vi "F5xxx_pq_set_harmonics.vi"(7 "max harms":i32=15, 8 "error in":errorcluster, 9 "channel":enum16{"PRI", "SEC"}(ring), 10 "harmonic list":T1[](array[typedef]), 11 "VISA in":refnum<visa-resource-name>) -> (0 "error out":errorcluster, 3 "VISA out":refnum<visa-resource-name>)   [LabVIEW 2013]
uses:
  F5xxx_pq_harmonic_def.ctl
  Fluke 5XXX Series Multicalibrators.lvlib
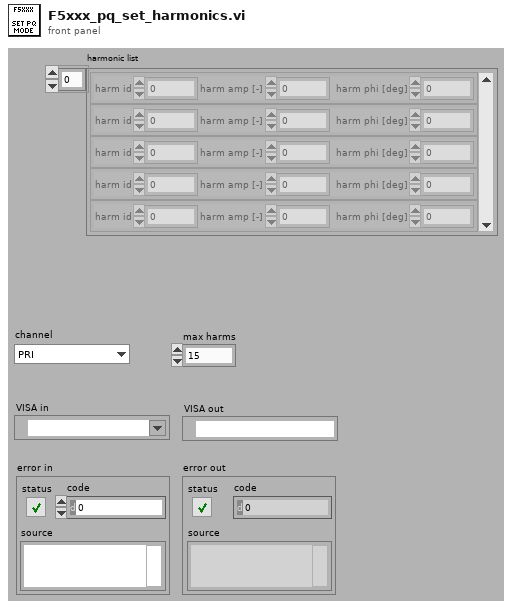
[diagram p1: front panel]
types:
  T1 = typedef "F5xxx_pq_harmonic_def.ctl" = cluster{"harm id":i32, "harm amp [-]":dbl, "harm phi [deg]":dbl}
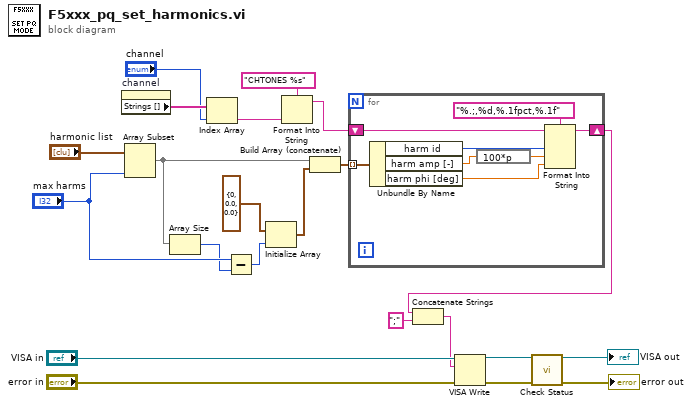
[diagram p0: block diagram]
diagram:
  n1 = property on="channel" class="Enum (strict)"() -> ("Strings []"=w8:string[])  [unwired: 2 in, 2 out]
  n2 = Array Subset(array="harmonic list", length="max harms") -> (w15:T1[])  [unwired: 1 in]
  n3 = Array Size(array=w15) -> (size(s)=w2:i32)
  n4 = Index Array(array=w8, index="channel") -> (element=w9:string)
  n5 = Subtract(x="max harms", y=w2) -> (x-y=w1:i32)
  n6 = Initialize Array(T1 {"harm id"=0, "harm amp [-]"=0.0, "harm phi [deg]"=0.0} ("Cluster"), w1) -> (w14:T1[])
  n7 = Format Into String(format string="CHTONES %s", w9) -> (resulting string=w10:string)  [unwired: 2 in, 1 out]
  n8 = Build Array (concatenate)(w15, w14) -> (w13:T1[])
  n9 = for {
    tunnel: w13 -> [w30] mode=indexing
    shift-right: [w23] -> w6
    shift-left: w10 -> [w24]
    n10 = Unbundle By Name(w30) -> ("harm id"=w29:i32, "harm amp [-]"=w28:dbl, "harm phi [deg]"=w26:dbl)
    n11 = expression code="100*p"(w28) -> (w27:dbl)
    n12 = Format Into String(format string="%.;,%d,%.1fpct,%.1f", initial string=w24, w29, w27, w26) -> (resulting string=w23:string)  [unwired: 1 in, 1 out]
  }
  n13 = Concatenate Strings(w6, ";" ("string")) -> (w5:string)
  n14 = VISA Write(VISA resource name="VISA in", write buffer=w5, error in (no error)="error in") -> (VISA resource name out=w20:refnum<visa-resource-name>, error out=w21:errorcluster)  [unwired: 1 out]
  n15 = call "Check Status.vi"("VISA resource name"=w20, "error in (no error)"=w21) -> ("VISA resource name out"=→"VISA out":refnum<visa-resource-name>, "error out"=→"error out":errorcluster)  [unwired: 12 in]
